vi "Default or Users ASCII or Unicode.vi"(0 "PDF Report IN":refnum<class "PDF Report Class.lvclass">, 7 "ASCII or Unicode IN":T1, 11 "error in (no error)":errorcluster) -> (4 "PDF Report OUT":refnum<class "PDF Report Class.lvclass">, 8 "ASCII or Unicode OUT":T1={"Type"=enum."ASCII", "Direction"=enum."Default"}, 15 "error out":errorcluster)   [LabVIEW 2019, in "Exaprom PDF.lvlib"]
doc: "Developed by Jean-Marc Simard\nCopyright © 2012, Exaprom Inc.\nAll rights reserved.\nLicense: BSD\n\nWith iTextSharp 4.1.6 (http://itextsharp.sourceforge.net)\nunder Mozilla Public License Version 1.1\n(http://www.mozilla.org/MPL/MPL-1.1.html)"
uses:
  Exaprom PDF.lvlib
  Controls/Text Controls/Unicode/Character type with Select.ctl
  Controls/Text Controls/Unicode/Writing direction with Select.ctl
  LV Class/PDF Report Class/PDF Report Class.lvclass
  C:/work/niobrara_lv/labview pdf writer fixing/LV Class/Fonts Class/Font Class.lvclass
  Controls/Text Controls/Unicode/ASCII or Unicode with Select.ctl
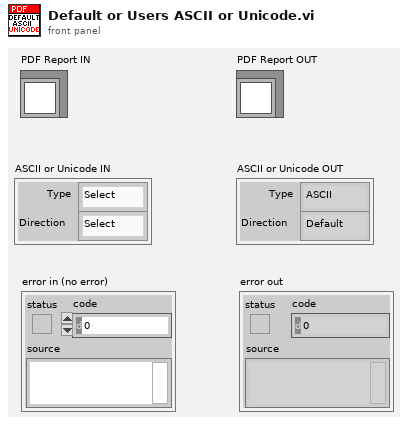
[diagram p1: front panel]
types:
  T1 = typedef "Exaprom PDF.lvlib/ASCII or Unicode with Select.ctl" = cluster{"Type":T2, "Direction":T3}
  T2 = typedef "Exaprom PDF.lvlib/Character type with Select.ctl" = enum16{"Select", "ASCII", "Unicode"}
  T3 = typedef "Exaprom PDF.lvlib/Writing direction with Select.ctl" = enum16{"Select", "Default", "NO BIDI", "LTR", "RTL"}
  T4 = typedef "ASCII or Unicode with Select.ctl" = cluster{"Type":T5, "Direction":T6}
  T5 = typedef "Character type with Select.ctl" = enum16{"Select", "ASCII", "Unicode"}
  T6 = typedef "Writing direction with Select.ctl" = enum16{"Select", "Default", "NO BIDI", "LTR", "RTL"}
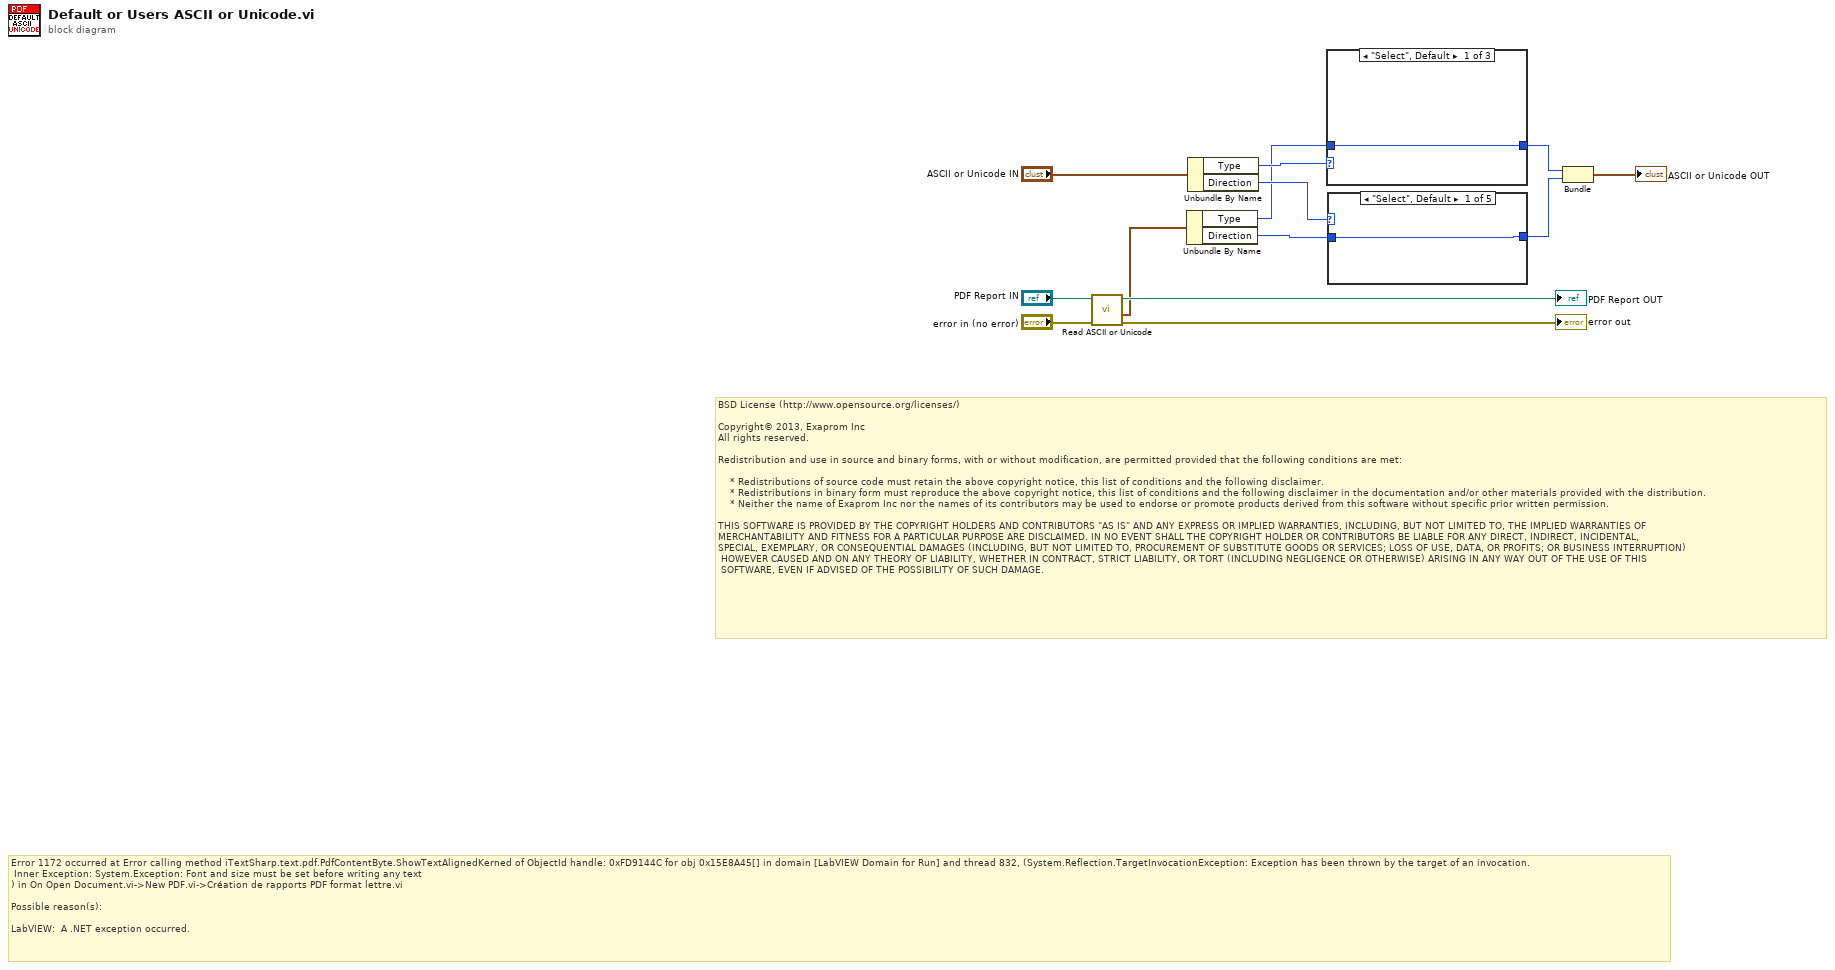
[diagram p0: block diagram]
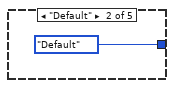
[diagram p2: hidden frame]
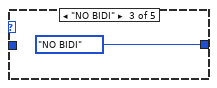
[diagram p3: hidden frame]
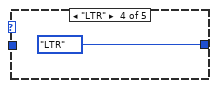
[diagram p4: hidden frame]
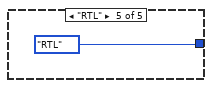
[diagram p5: hidden frame]
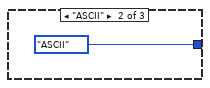
[diagram p6: hidden frame]
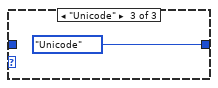
[diagram p7: hidden frame]
diagram:
  # "Error 1172 occurred at Error calling method iTextSharp.text.pdf.PdfContentByte.ShowTextAlignedKerned of ObjectId handle: 0xFD9144C for obj 0x15E8A45[] in domain [LabVIEW Domain for Run] and thread 832, (System.Reflection.TargetInvocationException: Exception has been thrown by the target of an invocation.\n\tInner Exception: System.Exception: Font and size must be set before writing any text\n) in On Open Document.vi->New PDF.vi->Création de rapports PDF format lettre.vi\n\nPossible reason(s):\n\nLabVIEW:  A .NET exception occurred."
  # "BSD License (http://www.opensource.org/licenses/)\n\nCopyright© 2013, Exaprom Inc\nAll rights reserved.\n\nRedistribution and use in source and binary forms, with or without modification, are permitted provided that the following conditions are met:\n\n    * Redistributions of source code must retain the above copyright notice, this list of conditions and the following disclaimer.\n    * Redistributions in binary form must reproduce the above copyright notice, this list of conditions and the following disclaimer in the documentation and/or other materials provided with the distribution.\n    * Neither the name of Exaprom Inc nor the names of its contributors may be used to endorse or promote products derived from this software without specific prior written permission.\n\nTHIS SOFTWARE IS PROVIDED BY THE COPYRIGHT HOLDERS AND CONTRIBUTORS \"AS IS\" AND ANY EXPRESS OR IMPLIED WARRANTIES, INCLUDING, BUT NOT LIMITED TO, THE IMPLIED WARRANTIES OF \nMERCHANTABILITY AND FITNESS FOR A PARTICULAR PURPOSE ARE DISCLAIMED. IN NO EVENT SHALL THE COPYRIGHT HOLDER OR CONTRIBUTORS BE LIABLE FOR ANY DIRECT, INDIRECT, INCIDENTAL,\nSPECIAL, EXEMPLARY, OR CONSEQUENTIAL DAMAGES (INCLUDING, BUT NOT LIMITED TO, PROCUREMENT OF SUBSTITUTE GOODS OR SERVICES; LOSS OF USE, DATA, OR PROFITS; OR BUSINESS INTERRUPTION)\n HOWEVER CAUSED AND ON ANY THEORY OF LIABILITY, WHETHER IN CONTRACT, STRICT LIABILITY, OR TORT (INCLUDING NEGLIGENCE OR OTHERWISE) ARISING IN ANY WAY OUT OF THE USE OF THIS\n SOFTWARE, EVEN IF ADVISED OF THE POSSIBILITY OF SUCH DAMAGE."
  n1 = call-dynamic "Read ASCII or Unicode.vi"("error in (no error)"="error in (no error)", "Font Class in"="PDF Report IN") -> ("error out"=→"error out":errorcluster, "ASCII or Unicode"=w2:T4, "Font Class out"=→"PDF Report OUT":refnum<class "PDF Report Class.lvclass">)  [unwired: 6 in, 1 out]
  n2 = Unbundle By Name(w2) -> ("Type"=w1:T5, "Direction"=w3:T6)
  n3 = Unbundle By Name("ASCII or Unicode IN") -> ("Type"=w8:T2, "Direction"=w7:T3)
  n4 = case shown="\"Select\", Default" w8 {
    tunnel: w1 -> [w14 _ _]
    tunnel: [w14 Character_type_with_Select."ASCII" ("Type") Character_type_with_Select."Unicode" ("Type")] -> w6
    frame "Select", Default {
    }
    frame "ASCII" {
    }
    frame "Unicode" {
    }
  }
  n5 = case shown="\"Select\", Default" w7 {
    tunnel: [w17 Writing_direction_with_Select."Default" ("Direction") Writing_direction_with_Select."NO BIDI" ("Direction") Writing_direction_with_Select."LTR" ("Direction") Writing_direction_with_Select."RTL" ("Direction")] -> w5
    tunnel: w3 -> [w17 _ _ _ _]
    frame "Select", Default {
    }
    frame "Default" {
    }
    frame "NO BIDI" {
    }
    frame "LTR" {
    }
    frame "RTL" {
    }
  }
  n6 = Bundle("Type"=w6, "Direction"=w5) -> (→"ASCII or Unicode OUT":cluster{"Type":T2, "Direction":T3})  [unwired: 1 in]
